vi "XML Script - Wire.vi"   [LabVIEW 2020]
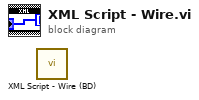
[diagram p0: block diagram]
diagram:
  n1 = call <vilib>:"XML Script - Wire (BD).vi"() -> ()  [unwired: 3 in, 3 out]
